vi "ScaleTo16Bit.vi"(8 "valid in":bool, 10 "factor":u16, 11 "val":fxp<+/-,18,1>) -> (0 "valid out":bool, 3 "16bit integer":i16)   [LabVIEW 2025]
uses:
  <vilib>/rvi/FXPMathLib/FxpConvert/subVIs/nifxpmath_Convert_SimConfig.ctl
  <vilib>/fxp/LVFixedPointQuantizationPolicyTypeDef.ctl
  <vilib>/fxp/LVFixedPointOverflowPolicyTypeDef.ctl
  <vilib>/rvi/FXPMathLib/FxpConvert/simVIs/DllFxpConvertTemp_sub.vi
  <vilib>/rvi/FXPMathLib/FxpInterpret/XNode/nifxpmath_Interpret.xnode
  <vilib>/rvi/FXPMathLib/FxpConvert/XNode/nifxpmath_Convert.xnode
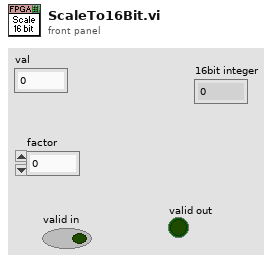
[diagram p1: front panel]
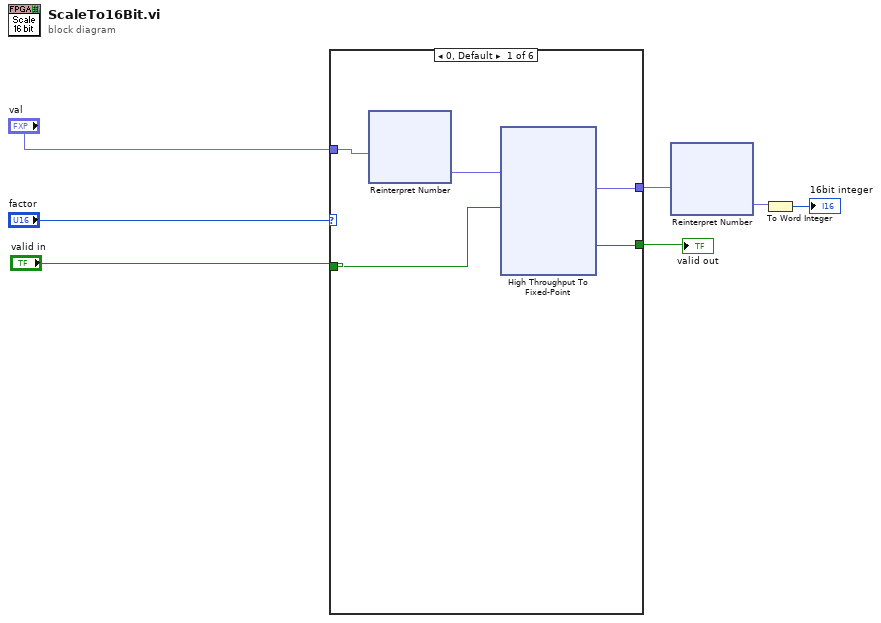
[diagram p0: block diagram]
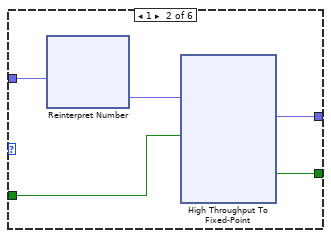
[diagram p2: hidden frame]
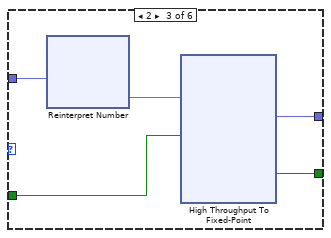
[diagram p3: hidden frame]
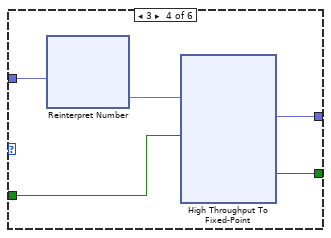
[diagram p4: hidden frame]
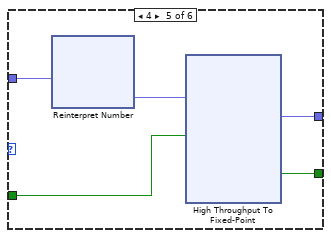
[diagram p5: hidden frame]
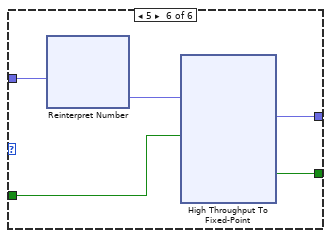
[diagram p6: hidden frame]
diagram:
  n1 = case shown="0, Default" "factor" {
    tunnel: "valid in" -> [w12 w39 w68 w97 w124 w155]
    tunnel: "val" -> [w9 w40 w69 w98 w127 w156]
    tunnel: [w10 w38 w66 w95 w125 w153] -> w5
    tunnel: [w11 w37 w67 w96 w126 w154] -> w1
    frame 0, Default {
      n2 = xnode "Reinterpret Number"("x"=w9) -> ("y"=w8:fxp<+/-,18,14>)
      n3 = xnode "High Throughput To Fixed-Point"("x"=w8, "input valid"=w12) -> ("y"=w11:fxp<+/-,16,14>, "output valid"=w10:bool)  [unwired: 1 in, 1 out]
    }
    frame 1 {
      n4 = xnode "Reinterpret Number"("x"=w40) -> ("y"=w41:fxp<+/-,18,15>)
      n5 = xnode "High Throughput To Fixed-Point"("x"=w41, "input valid"=w39) -> ("y"=w37:fxp<+/-,16,14>, "output valid"=w38:bool)  [unwired: 1 in, 1 out]
    }
    frame 2 {
      n6 = xnode "Reinterpret Number"("x"=w69) -> ("y"=w70:fxp<+/-,18,16>)
      n7 = xnode "High Throughput To Fixed-Point"("x"=w70, "input valid"=w68) -> ("y"=w67:fxp<+/-,16,14>, "output valid"=w66:bool)  [unwired: 1 in, 1 out]
    }
    frame 3 {
      n8 = xnode "Reinterpret Number"("x"=w98) -> ("y"=w99:fxp<+/-,18,17>)
      n9 = xnode "High Throughput To Fixed-Point"("x"=w99, "input valid"=w97) -> ("y"=w96:fxp<+/-,16,14>, "output valid"=w95:bool)  [unwired: 1 in, 1 out]
    }
    frame 4 {
      n10 = xnode "Reinterpret Number"("x"=w127) -> ("y"=w128:fxp<+/-,18,18>)
      n11 = xnode "High Throughput To Fixed-Point"("x"=w128, "input valid"=w124) -> ("y"=w126:fxp<+/-,16,14>, "output valid"=w125:bool)  [unwired: 1 in, 1 out]
    }
    frame 5 {
      n12 = xnode "Reinterpret Number"("x"=w156) -> ("y"=w157:fxp<+/-,18,19>)
      n13 = xnode "High Throughput To Fixed-Point"("x"=w157, "input valid"=w155) -> ("y"=w154:fxp<+/-,16,14>, "output valid"=w153:bool)  [unwired: 1 in, 1 out]
    }
  }
  "valid out" <- w5
  n14 = xnode "Reinterpret Number"("x"=w1) -> ("y"=w4:fxp<+/-,16,16>)
  n15 = To Word Integer(number=w4) -> (16bit integer=→"16bit integer":i16)
